vi "Add.vi"(8 "error in (no error)":errorcluster caption="错误输入（无错误）", 10 "anything":variant caption="任何数据", 11 "ArrayListClass 输入":refnum<class "ArrayListClass.lvclass"> caption="DNL_LabVIEW Object in") -> (0 "error out":errorcluster caption="错误输出", 3 "ArrayListClass 输出":refnum<class "ArrayListClass.lvclass"> caption="DNL_LabVIEW Object out")   [LabVIEW 2012, in "ArrayListClass.lvclass"]
uses:
  ArrayListClass.lvclass
  ArrayListClass.lvclass/ArrayListClass.ctl
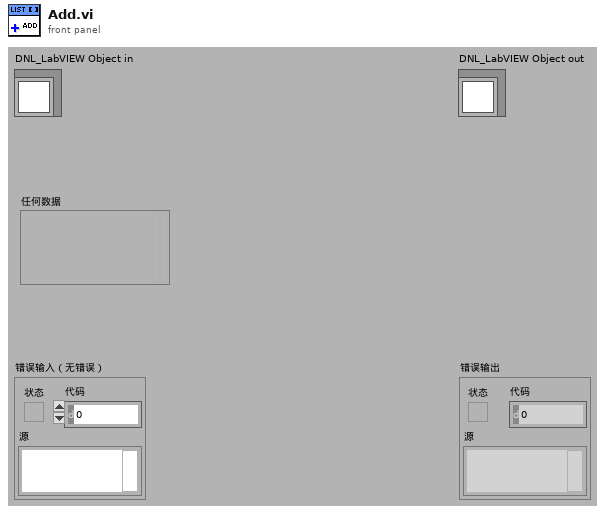
[diagram p1: front panel]
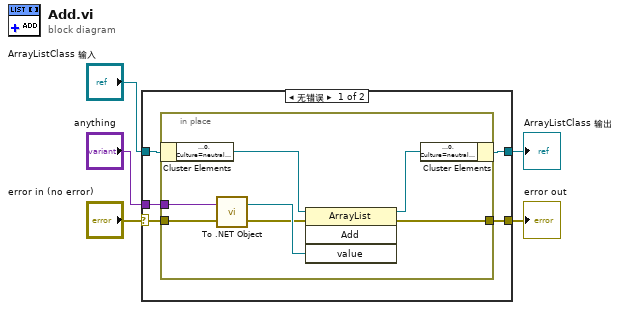
[diagram p0: block diagram]
diagram:
  n1 = case shown="无错误" "error in (no error)" {
    selector: "error in (no error)" -> [w7 w19]
    tunnel: [w6 w19] -> w4
    tunnel: [w8 w18] -> w2
    tunnel: "ArrayListClass 输入" -> [w10 w18]
    tunnel: "anything" -> [w9 _]
    frame No Error {
      n2 = in-place {
        in-place-border: w9 -> [w14]
        in-place-border: w7 -> [w12]
        in-place-border: [w13] -> w6
        n3 = in-place-cluster #1(w10) -> ("ArrayList"=w17:refnum<k24>)
        n4 = call <vilib>:"To .NET Object.vi"("error in (no error)"=w12, "anything"=w14) -> ("error out"=w11:errorcluster, ".NET object"=w15:refnum<k24>)
        n5 = invoke class="ArrayList" method="Add"(reference=w17, error in=w11, "value"=w15) -> (reference out=w16:refnum<k24>, error out=w13:errorcluster)  [unwired: 1 in, 2 out]
        n6 = in-place-cluster #1("ArrayList"=w16) -> (w8:refnum<class "ArrayListClass.lvclass">)
      }
    }
    frame Error {
    }
  }
  "error out" <- w4
  "ArrayListClass 输出" <- w2
